vi "Init Hardware.vi"(8 "error in (no error)":errorcluster, 11 "DAQmx Digitizer in":refnum<class "DAQmx Synthesizer.lvclass">) -> (0 "error out":errorcluster, 3 "DAQmx Digitizer out":refnum<class "DAQmx Synthesizer.lvclass">)   [LabVIEW 2019, in "DAQmx Synthesizer.lvclass"]
uses:
  DAQmx Synthesizer.lvclass
  C:/github/NHMFL_Core/Libraries/Instruments/Pulse Driver/Pulse Driver.lvclass
  DAQmx Synthesizer.lvclass/DAQmx Synthesizer.ctl
  Instruments/Pulse Driver/Pulse Driver.lvclass/Pulse Driver.ctl
  <vilib>/DAQmx/write.llb/DAQmx Write (Analog 1D Wfm NChan NSamp).vi
  Instruments/Pulse Driver/Read Pretrigger samples.vi
  Instruments/Pulse Driver/Read Samples per channel.vi
  Instruments/Pulse Driver/Write t0.vi
  Instruments/Pulse Driver/Write dt.vi
  Instruments/Pulse Driver/Write Set timing from UI.vi
  <vilib>/DAQmx/create/channels.llb/DAQmx Create Channel (AO-Voltage-Basic).vi
  <vilib>/DAQmx/configure/timing.llb/DAQmx Timing (Sample Clock).vi
  <vilib>/DAQmx/configure/trigger.llb/DAQmx Start Trigger (Digital Edge).vi
  <vilib>/DAQmx/miscellaneous.llb/DAQmx Fill In Error Info.vi
  <resource>/objmgr/daqmx.rc
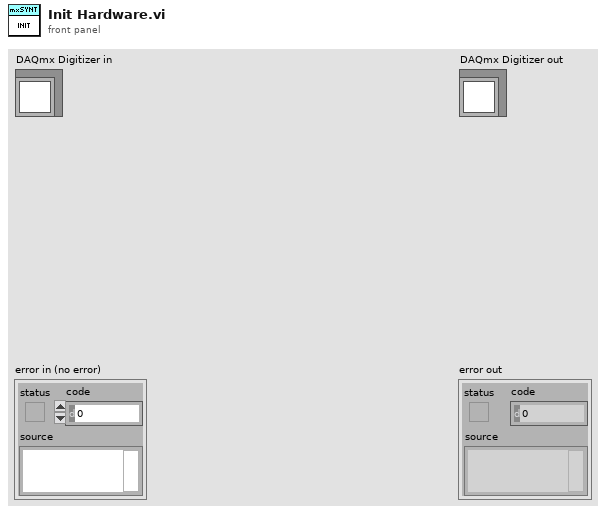
[diagram p1: front panel]
types:
  T1 = typedef "DAQmx Synthesizer Configuration.ctl" = cluster{"Ranges":dbl[], "Channel names":string[], "Output channels":string, "File Path Control":path}
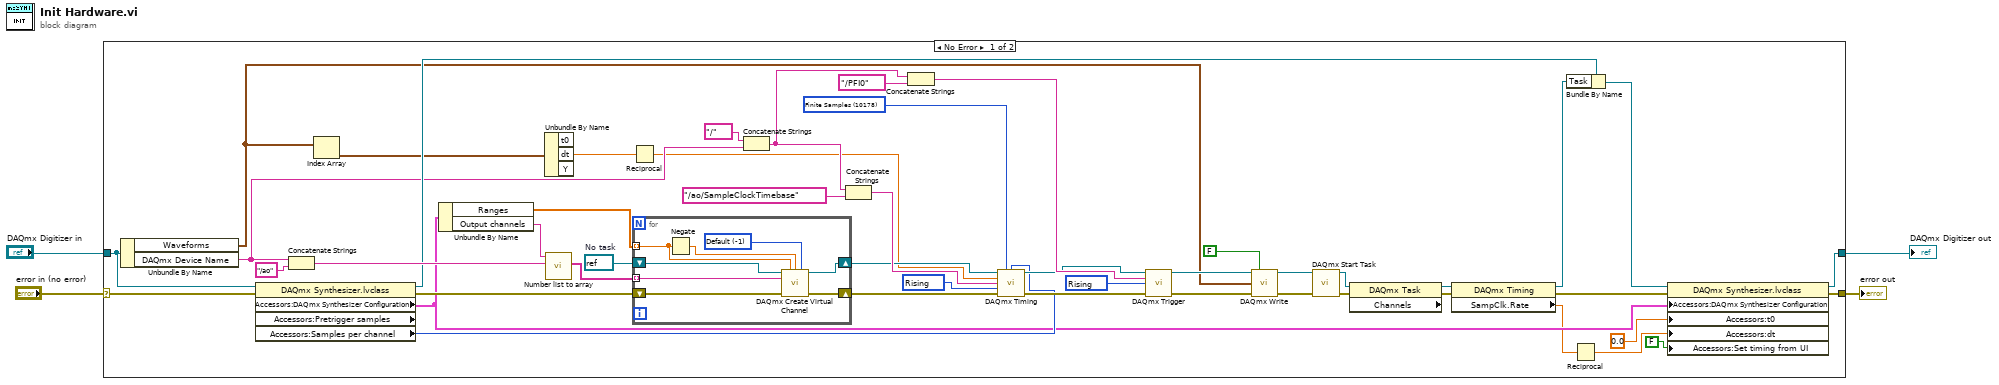
[diagram p0: block diagram]
diagram:
  n1 = case shown="No Error" "error in (no error)" {
    selector: "error in (no error)" -> [w33 w62]
    tunnel: [w34 w62] -> w3
    tunnel: [w35 w61] -> w1
    tunnel: "DAQmx Digitizer in" -> [w31 w61]
    frame No Error {
      w37 = refnum<k21> refnum  # No task
      w44 = 10280 items=["Rising"=10280, "Falling"=10171] ("active edge")
      w45 = 10178 items=["Finite Samples"=10178, "Continuous Samples"=10123, "Hardware Timed Single Point"=12522] ("sample mode")
      w52 = 10280 items=["Rising"=10280, "Falling"=10171] ("edge")
      n2 = Unbundle By Name(w31) -> ("Waveforms"=w8:waveform(dbl)[], "DAQmx Device Name"=w18:tag)
      n3 = property class="DAQmx Synthesizer.lvclass" props=["Accessors:DAQmx Synthesizer Configuration", "Accessors:Pretrigger samples", "Accessors:Samples per channel"](reference=w31, error in=w33) -> (reference out=w30:refnum<class "DAQmx Synthesizer.lvclass">, error out=w32:errorcluster, "Accessors:DAQmx Synthesizer Configuration"=w26:T1, "Accessors:Samples per channel"=w27:i32)  [unwired: 1 out]
      n4 = Concatenate Strings(w18, "/ao" ("string")) -> (w38:string)
      n5 = Index Array(array=w8) -> (element=w15:waveform(dbl))  [unwired: 1 in]
      n6 = Unbundle By Name(w26) -> ("Ranges"=w25:dbl[], "Output channels"=w40:string)
      n7 = Unbundle By Name(w15) -> ("dt"=w14:dbl)  [unwired: 2 out]
      n8 = call "Number list to array.vi"("Full names prefix"=w38, "Number list"=w40) -> ("Full names"=w36:string[])  [unwired: 8 in, 1 out]
      n9 = Reciprocal(x=w14) -> (1/x=w13:dbl)
      n10 = for {
        tunnel: w36 -> [w60] mode=indexing
        tunnel: w25 -> [w58] mode=indexing
        shift-right: [w55] -> w51
        shift-left: w32 -> [w59]
        shift-right: [w56] -> w24
        shift-left: w37 -> [w53]
        w54 = -1 items=["Default"=-1, "RSE"=10083, "NRSE"=10078, "Differential"=10106, "Pseudodifferential"=12529] ("input terminal configuration")
        n11 = Negate(x=w58) -> (-x=w57:dbl)
        n12 = call-poly <vilib>:"DAQmx Create Virtual Channel.vi"("task in"=w53, "maximum value"=w58, "minimum value"=w57, "output terminal configuration"=w54, "physical channels"=w60, "error in"=w59) -> ("task out"=w56:refnum<k21>, "error out"=w55:errorcluster)  [unwired: 8 in]
      }
      n13 = Concatenate Strings(tag "/" ("string"), w18) -> (w16:string)
      n14 = Concatenate Strings(w16, tag "/ao/SampleClockTimebase" ("string")) -> (w43:string)
      n15 = Concatenate Strings(w16, tag "/PFI0" ("string")) -> (w49:string)
      n16 = call-poly <vilib>:"DAQmx Timing.vi"("task/channels in"=w24, "sample mode"=w45, "samples per channel"=w27, "rate"=w13, "source"=w43, "active edge"=w44, "error in"=w51) -> ("task out"=w47:refnum<k21>, "error out"=w48:errorcluster)  [unwired: 7 out]
      n17 = call-poly <vilib>:"DAQmx Trigger.vi"("task/channels in"=w47, "source"=w49, "edge"=w52, "error in"=w48) -> ("task out"=w12:refnum<k21>, "error out"=w10:errorcluster)  [unwired: 10 out]
      n18 = call-poly <vilib>:"DAQmx Write.vi"("task/channels in"=w12, "auto start"=FALSE, "data"=w8, "error in"=w10) -> ("task out"=w11:refnum<k21>, "error out"=w9:errorcluster)  [unwired: 9 in, 1 out]
      n19 = call <vilib>:"DAQmx Start Task.vi"("task/channels in"=w11, "error in"=w9) -> ("task out"=w42:refnum<k21>, "error out"=w41:errorcluster)  [unwired: 12 out]
      n20 = property class="DAQmx Task" props=["Channels"](reference=w42, error in=w41) -> (reference out=w29:refnum<k21>, error out=w28:errorcluster)  [unwired: 1 out]
      n21 = property class="DAQmx Timing"(reference=w29, error in=w28) -> (reference out=w5:refnum<k21>, error out=w22:errorcluster, "SampClk.Rate"=w23:dbl)
      n22 = Bundle By Name(cluster=w30, "Task"=w5) -> (w50:refnum<class "DAQmx Synthesizer.lvclass">)
      n23 = Reciprocal(x=w23) -> (1/x=w21:dbl)
      n24 = property class="DAQmx Synthesizer.lvclass"(reference=w50, error in=w22, "Accessors:DAQmx Synthesizer Configuration"=w26, "Accessors:t0"=0.0, "Accessors:dt"=w21, "Accessors:Set timing from UI"=FALSE ("Set timing from UI")) -> (reference out=w35:refnum<class "DAQmx Synthesizer.lvclass">, error out=w34:errorcluster)
    }
    frame Error {
    }
  }
  "error out" <- w3
  "DAQmx Digitizer out" <- w1
